vi "TAT_Login Screen.vi"(8 "Error In":errorcluster, 10 "Password":string, 11 "User Name":string(combo)) -> (0 "error out":errorcluster, 1 "Level":i32, 2 "Login Done":bool, 3 "User Name Out":string(combo))   [LabVIEW 2017]
uses:
  <vilib>/Utility/config.llb/Read Key (String).vi
  <vilib>/Utility/config.llb/Read Key (I32).vi
  <vilib>/Utility/config.llb/NI_LVConfig.lvlib
panel:
  in  "Cancel":bool
  in  "OK Button":bool
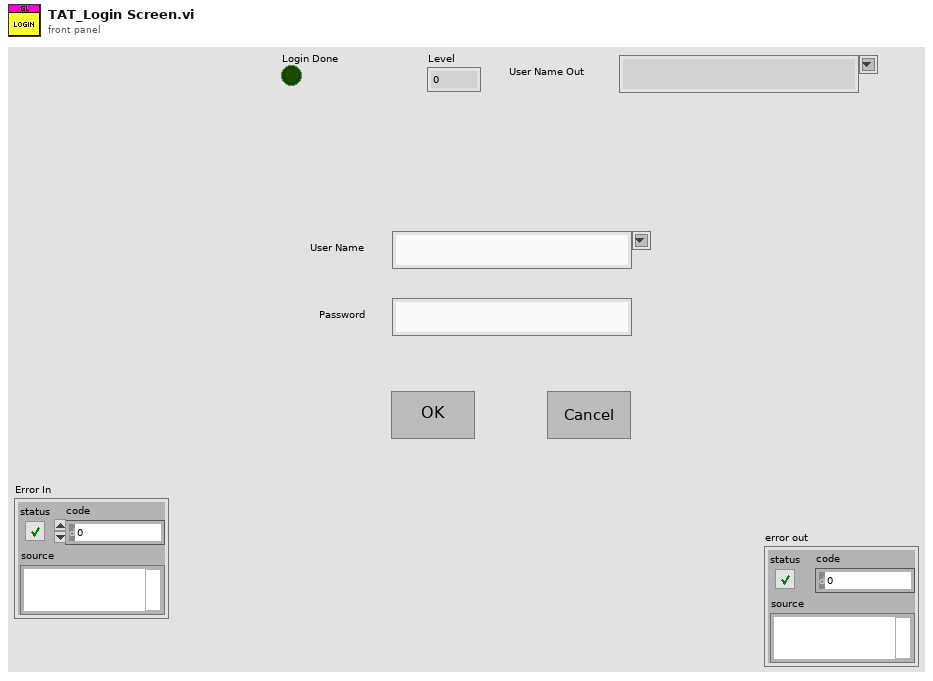
[diagram p1: front panel]
types:
  T1 = enum32{"invalid app kind", "Development System", "Run Time System", "Student Edition", "Embedded LabVIEW", "Evaluation", "Custom"}
  T2 = typedef "NI_LVConfig.lvlib/Config Data RefNum.ctl" = refnum<k1>
  T3 = enum32{"Invalid", "Standard", "Closed", "Hidden", "Minimized", "Maximized"}
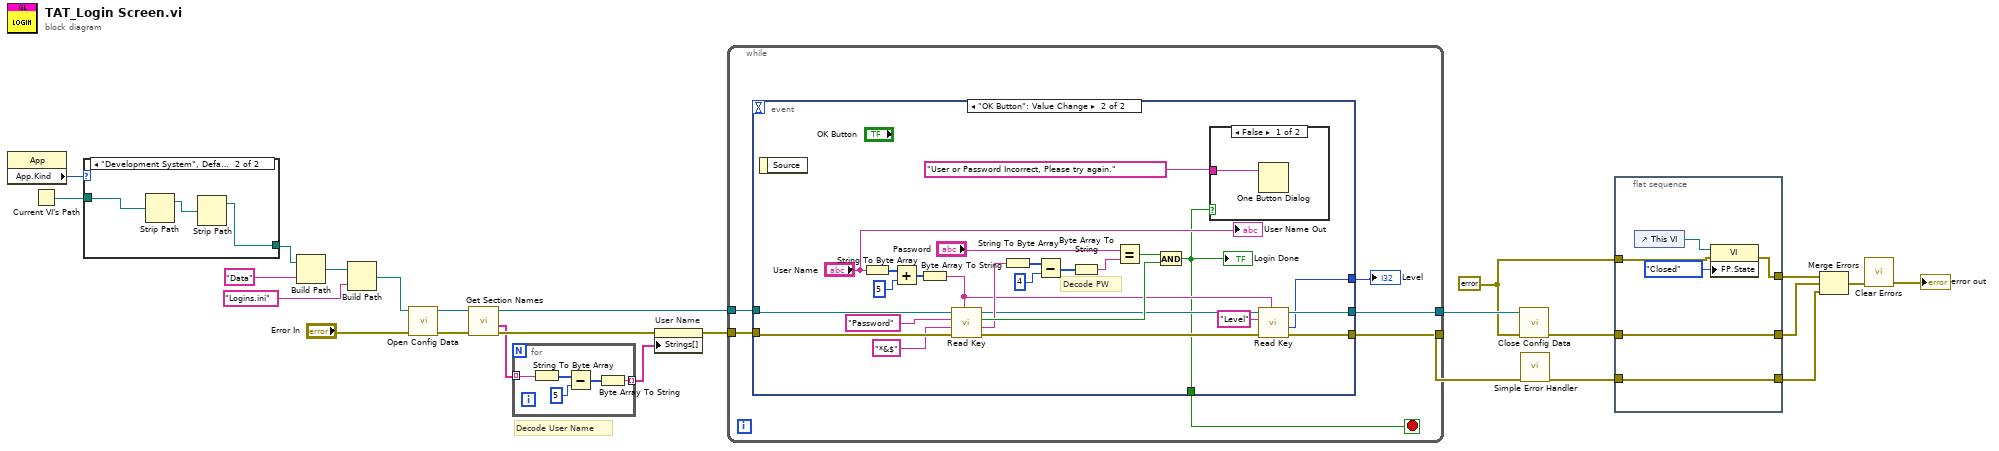
[diagram p0: block diagram]
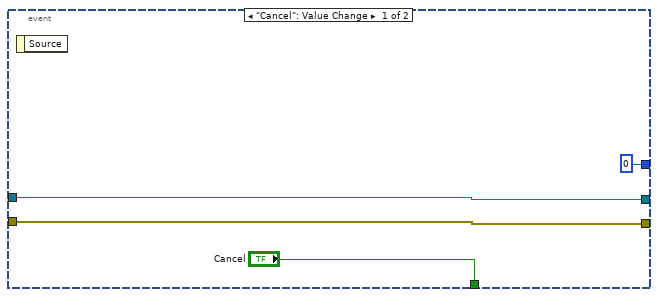
[diagram p2: hidden frame]
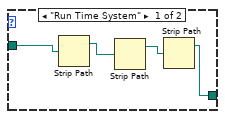
[diagram p4: hidden frame]
diagram:
  w15 = errorcluster {"status"=FALSE, "code"=0, "source"=""} ("error in (no error)")
  # "Decode User Name"
  n1 = property class="App"() -> ("App.Kind"=w23:T1)  [unwired: 2 in, 2 out]
  n2 = Current VI's Path() -> (path=w24:path)
  n3 = case shown="\"Development System\", Default" w23 {
    tunnel: w24 -> [w27 w31]
    tunnel: [w26 w30] -> w21
    frame "Run Time System" {
      n4 = Strip Path(path=w27) -> (stripped path=w29:path)  [unwired: 1 out]
      n5 = Strip Path(path=w29) -> (stripped path=w28:path)  [unwired: 1 out]
      n6 = Strip Path(path=w28) -> (stripped path=w26:path)  [unwired: 1 out]
    }
    frame "Development System", Default {
      n7 = Strip Path(path=w31) -> (stripped path=w32:path)  [unwired: 1 out]
      n8 = Strip Path(path=w32) -> (stripped path=w30:path)  [unwired: 1 out]
    }
  }
  n9 = Build Path(base path=w21, name or relative path="Data") -> (appended path=w22:path)
  n10 = Build Path(base path=w22, name or relative path="Logins.ini") -> (appended path=w20:path)
  n11 = call <vilib>:"Open Config Data.vi"("error in (no error)"="Error In", "configuration file path"=w20) -> ("error out"=w6:errorcluster, "refnum"=w7:T2)  [unwired: 7 in, 1 out]
  n12 = call <vilib>:"Get Section Names.vi"("error in (no error)"=w6, "refnum"=w7) -> ("error out"=w4:errorcluster, "section names"=w2:string[], "refnum out"=w5:T2)  [unwired: 7 in]
  n13 = for {
    tunnel: w2 -> [w37] mode=indexing
    tunnel: [w33] -> w1 mode=indexing
    n14 = String To Byte Array(string=w37) -> (unsigned byte array=w36:u8[])
    n15 = Subtract(x=w36, y=u8 5) -> (x-y=w34:u8[])
    n16 = Byte Array To String(unsigned byte array=w34) -> (string=w33:string)
  }
  n17 = property on="User Name" class="CmbBox"(error in=w4, "Strings[]"=w1) -> (error out=w3:errorcluster)  [unwired: 1 in, 1 out]
  n18 = while {
    tunnel: [w42] -> w17
    tunnel: w5 -> [w41]
    tunnel: [w40] -> w16
    tunnel: w3 -> [w39]
    stop <- w43 stop-if-true
    n19 = event shown="[1] \"OK Button\": Value Change" {
      selector: _ -> [_ _]
      dyn-events: _ -> [_ _]
      timeout: _ -> [_ _]
      tunnel: ["Cancel" w49] -> w43
      tunnel: [w46 w53] -> w42
      tunnel: w41 -> [w46 w72]
      tunnel: [w45 w52] -> w40
      tunnel: w39 -> [w45 w71]
      tunnel: [0 ("value") w50] -> w38
      event "Cancel": Value Change {
        n20 = event-data() -> ()  [unwired: 1 in, 1 out]
      }
      event "OK Button": Value Change {
        # "Decode PW"
        n21 = event-data() -> ()  [unwired: 1 in, 1 out]
        n22 = String To Byte Array(string="User Name") -> (unsigned byte array=w60:u8[])
        n23 = Add(x=w60, y=u8 5) -> (x+y=w58:u8[])
        n24 = Byte Array To String(unsigned byte array=w58) -> (string=w56:string)
        n25 = call-poly <vilib>:"Read Key.vi"("section"=w56, "error in (no error)"=w71, "default value"="*&$", "key"="Password", "refnum"=w72) -> ("error out"=w55:errorcluster, "value"=w65:string, "found?"=w67:bool, "refnum out"=w54:T2)  [unwired: 3 in]
        n26 = String To Byte Array(string=w65) -> (unsigned byte array=w64:u8[])
        n27 = Subtract(x=w64, y=u8 4) -> (x-y=w62:u8[])
        n28 = Byte Array To String(unsigned byte array=w62) -> (string=w61:string)
        n29 = Equal?(x="Password", y=w61) -> (x = y?=w68:bool)
        n30 = And(x=w68, y=w67) -> (x .and. y?=w49:bool)
        "Login Done" <- w49
        n31 = case shown="False" w49 {
          tunnel: "User or Password Incorrect, Please try again." -> [w73 _]
          frame False {
            n32 = One Button Dialog(message=w73) -> ()  [unwired: 1 in, 1 out]
          }
          frame True {
          }
        }
        n33 = call-poly <vilib>:"Read Key.vi"("section"=w56, "error in (no error)"=w55, "key"="Level", "refnum"=w54) -> ("error out"=w52:errorcluster, "value"=w50:i32, "refnum out"=w53:T2)  [unwired: 4 in, 1 out]
        "User Name Out" <- "User Name"
      }
    }
    "Level" <- w38
  }
  n34 = call <vilib>:"Close Config Data.vi"("error in (no error)"=w15, "refnum"=w17) -> ("error out"=w10:errorcluster)  [unwired: 8 in, 1 out]
  n35 = call <vilib>:"Simple Error Handler.vi"("error in (no error)"=w16) -> ("error out"=w8:errorcluster)  [unwired: 4 in, 4 out]
  n36 = flat-sequence {
    tunnel: w15 -> [w77]
    tunnel: [w76] -> w14
    tunnel: [w75] -> w11
    tunnel: w10 -> [w75]
    tunnel: [w74] -> w9
    tunnel: w8 -> [w74]
    frame #0 {
      n37 = control-ref of="This VI"() -> (w79:refnum<vi>)
      n38 = property class="VI"(reference=w79, error in=w77, "FP.State"=T3."Closed" ("Front Panel Window:State")) -> (error out=w76:errorcluster)  [unwired: 1 out]
    }
  }
  n39 = Merge Errors(w14, w11, w9) -> (w13:errorcluster)
  n40 = call <vilib>:"Clear Errors.vi"("error in (no error)"=w13) -> ("error out"=→"error out":errorcluster)  [unwired: 5 in, 1 out]
